vi "!DB_editor_Main.vi"(8 "error in (no error)":errorcluster, 11 "DB-editor in":refnum<class "DB-editor.lvclass">) -> (0 "error out":errorcluster, 3 "DB-editor out":refnum<class "DB-editor.lvclass">)   [LabVIEW 2020, in "Sgraph_lib_V1.lvlib" / "DB-editor.lvclass"]
doc: "Andre Koelewijn, 18 aug 2021\n\nDatabase properties editor application.\nOnly one instance of this VI should run, and only for administrative purposes.\n(only to be used to change settings)"
uses:
  DB-editor.lvclass
  Common/controls/typedef_com_TagProp.ctl
  FAMM/controls/Typedef_Gviewer_TagsUnits.ctl
  Gserver/controls/Typedef_QueryType.ctl
  DB-editor.lvclass/DB-editor.ctl
  Builds/Sgraph_lib_V1.lvlib
  FAMM/FAMM.lvclass
  Gserver/Gserver.lvclass
panel:
  in  "TAGprop":T1 {"TagFunc" format="%08x"; "RangeL" format="%.2f"; "RangeH" format="%.2f"}
  in  "Cancel":bool
  in  "Save":bool
  out "Qtype":string
  out "TAG":string
  in  "Ring":u16(ring)
  out "37x37":picture
  # "Database Editor"
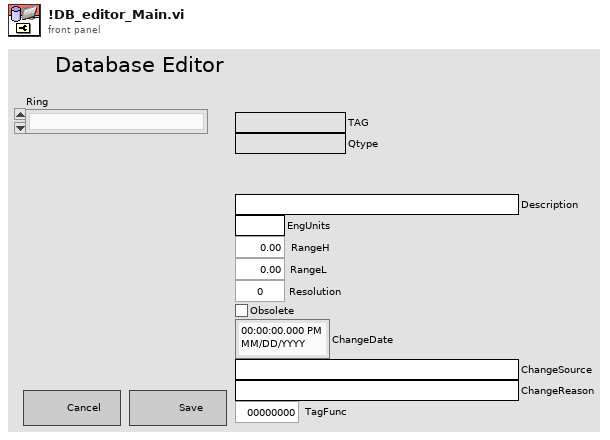
[diagram p1: front panel]
types:
  T1 = typedef "Sgraph_lib_V1.lvlib/typedef_com_TagProp.ctl" = cluster{"Description":string, "EngUnits":string, "RangeH":dbl, "RangeL":dbl, "Resolution":i32, "Obsolete":bool, "ChangeDate":timestamp, "ChangeSource":string, "ChangeReason":string, "TagFunc":u32}
  T2 = typedef "Sgraph_lib_V1.lvlib/FAMM.lvclass/Typedef_Gviewer_TagsUnits.ctl" = cluster{"PAQ_TAGs":string[], "WAQ_TAGs":string[], "EAQ_TAGs":string[], "PAQtagProps":T1[], "WAQtagProps":T1[], "EAQtagProps":T1[]}
  T3 = typedef "Sgraph_lib_V1.lvlib/Gserver.lvclass/Typedef_QueryType.ctl" = enum16{"Subscribe", "SubscribeNetw", "DataRequest", "RequestAllTags", "RequestIniPath", "FAMMstarted", "SetClientOptions", "GviewerUpdate", "OpenNewGraph", "CloseClient", "CloseAllClients", "Close Gserver", "OpenMemoryMap", "MeMapDataRequest", "MeMapDataResponse", "OpenDBeditor", "CheckDBeditorRunning", "StoppedDBeditor", "SaveDB_TAGpropRecord", "ConfirmDB_TAGpropSave", "GetXconstraints", "OpenNewNetworkGraph"}
  T4 = enum8{"Enabled", "Disabled", "Disabled and Grayed Out"}
  T5 = typedef "Typedef_Gserver-Replies.ctl" = cluster{"ServerActions":T6, "data":variant, "Source":string, "Time Stamp":timestamp}
  T6 = typedef "Sgraph_lib_V1.lvlib/Gviewer.lvclass/Typedef_ServerActions.ctl" = enum16{"GraphUpdate", "SendAllTags", "SendIniPath", "SetGeneralOptions", "EditTagsOpen", "EditTagsPresetSave", "EditTagsPresetLoad", "EditTagsClose", "NewTagSelection", "AutoScale", "DBeditStatus", "DBsaveConfirm", "GetXconstraints", "ExitGraph"}
  T7 = typedef "Sgraph_lib_V1.lvlib/DBAL.lvclass/DBAL_TAGprops.ctl" = T8[]
  T8 = typedef "Sgraph_lib_V1.lvlib/DBAL.lvclass/DBAL_TAGpropEdit.ctl" = cluster{"TAG":string, "Qtype":string, "TAGprop":T1}
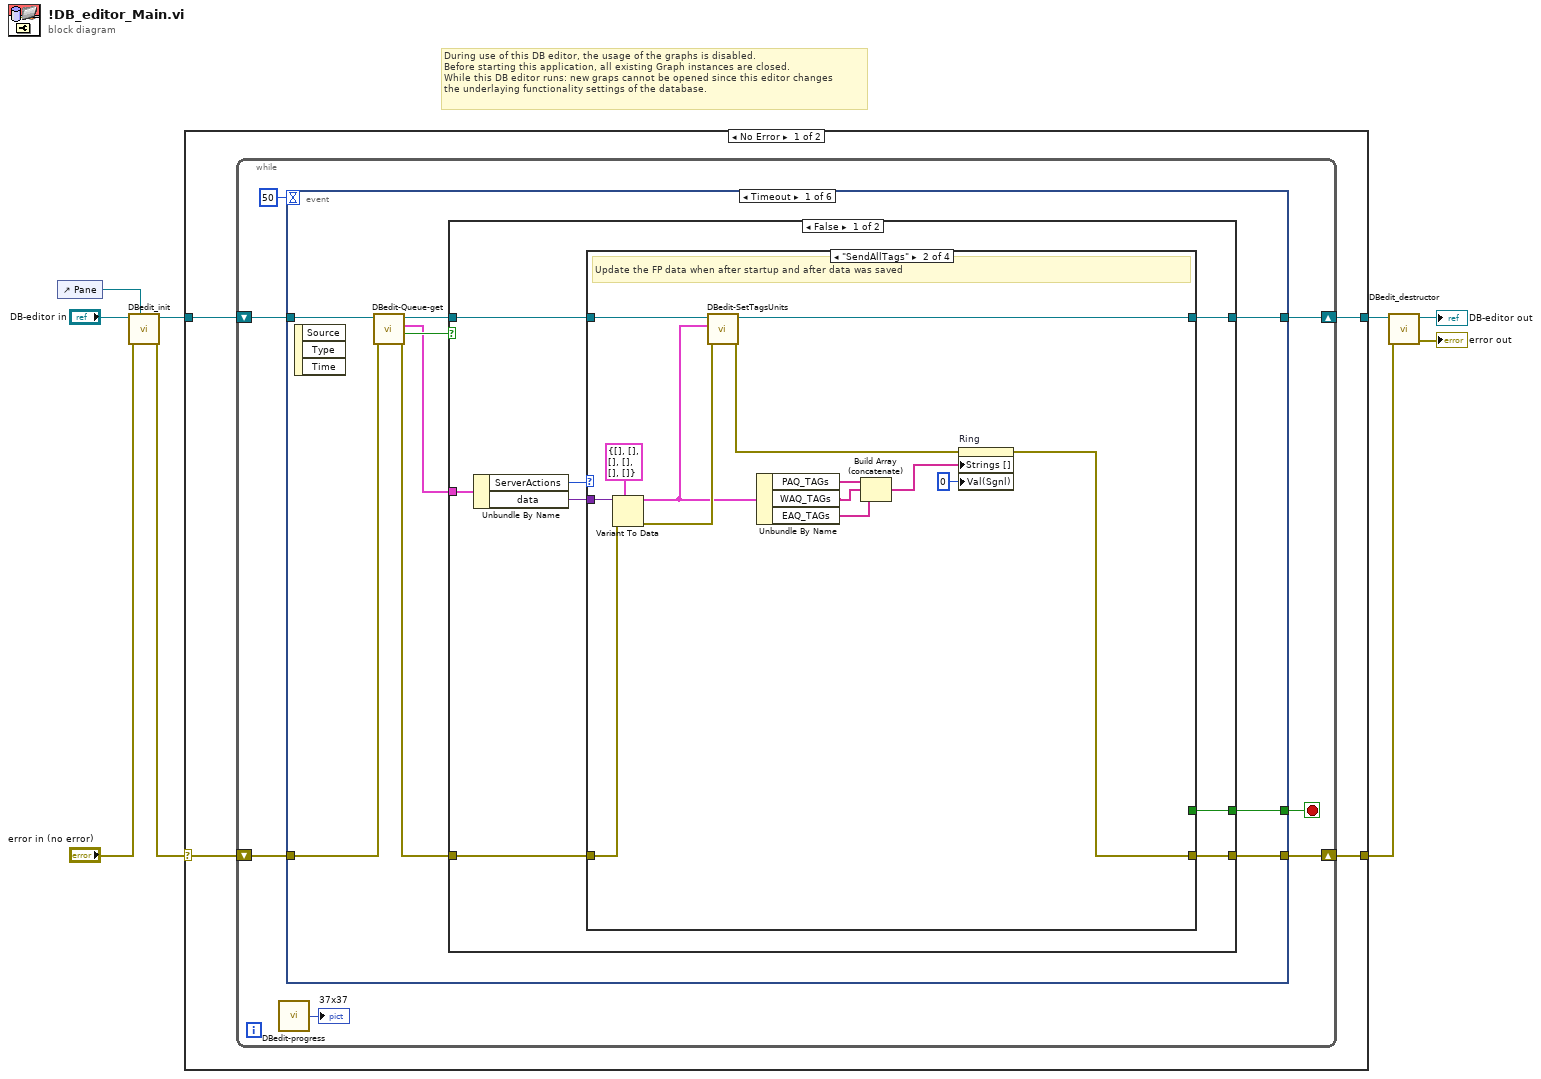
[diagram p0: block diagram]
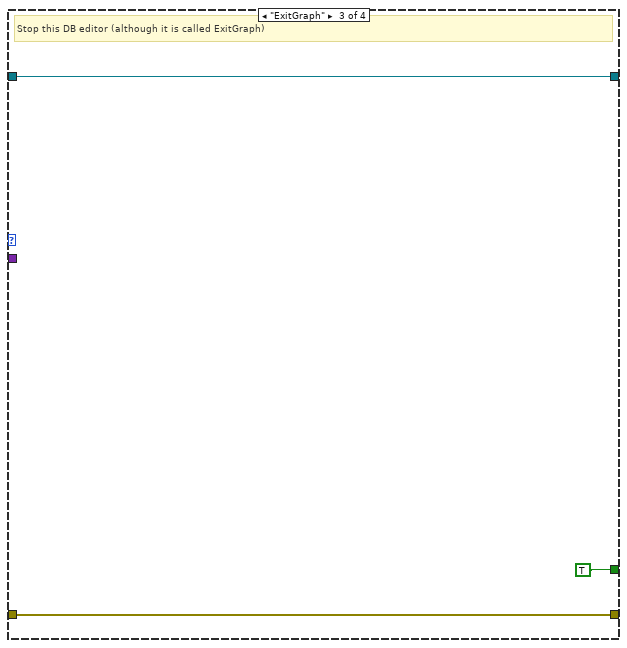
[diagram p3: hidden frame]
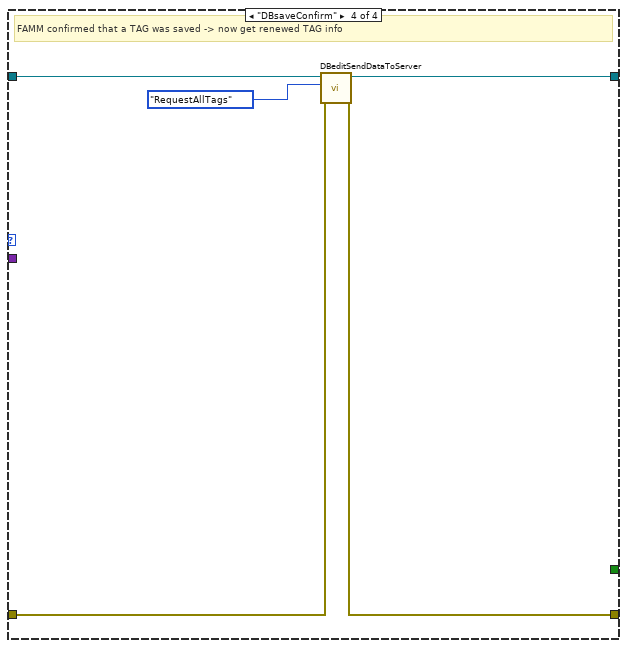
[diagram p4: hidden frame]
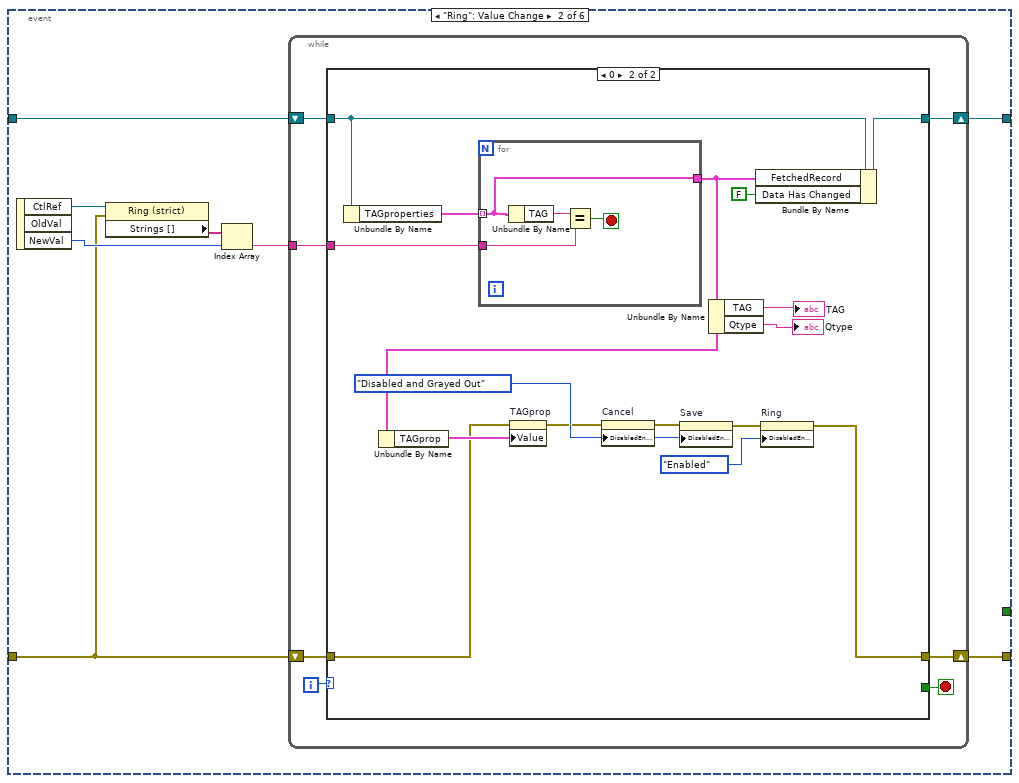
[diagram p6: hidden frame]
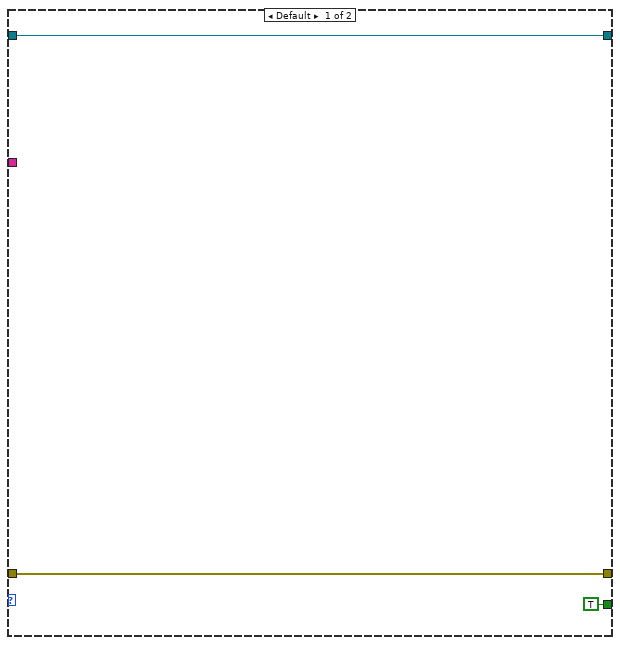
[diagram p7: hidden frame]
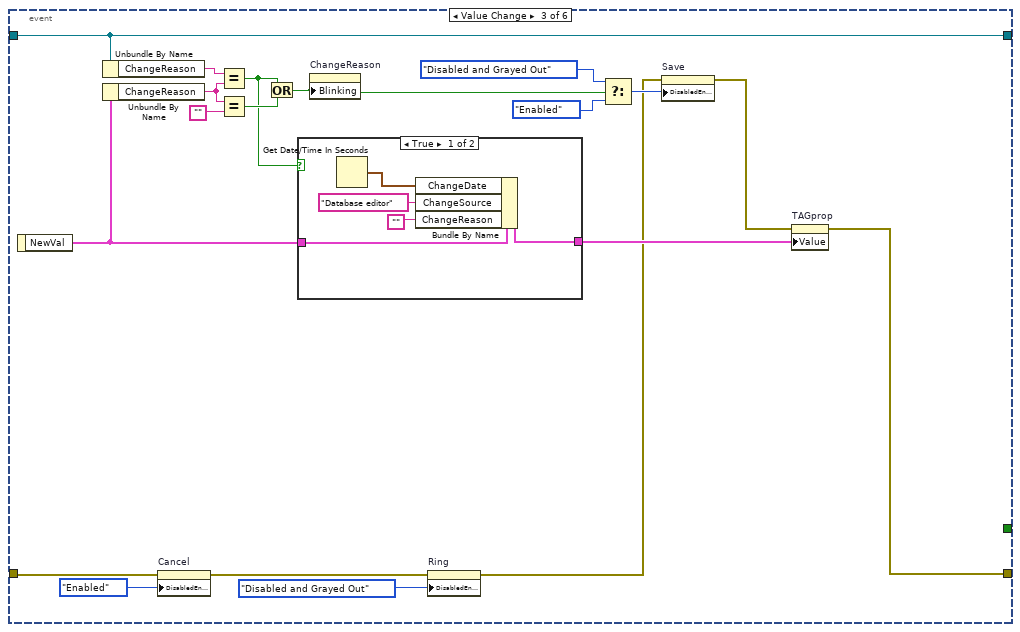
[diagram p8: hidden frame]
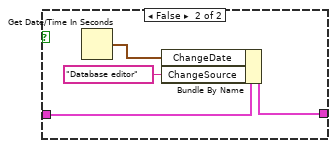
[diagram p9: hidden frame]
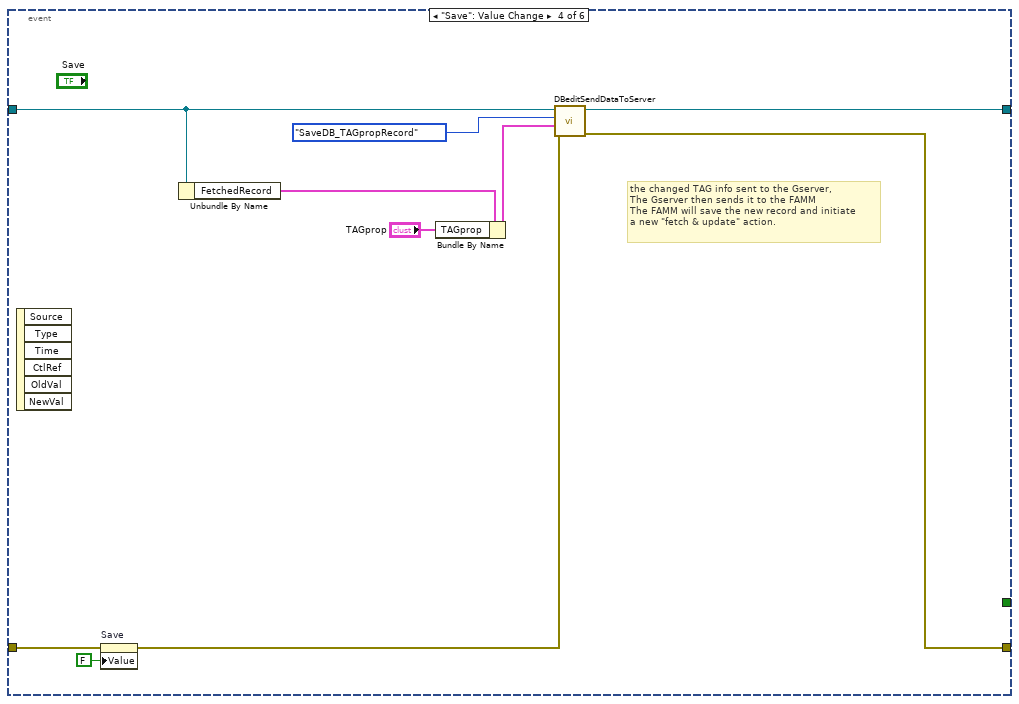
[diagram p10: hidden frame]
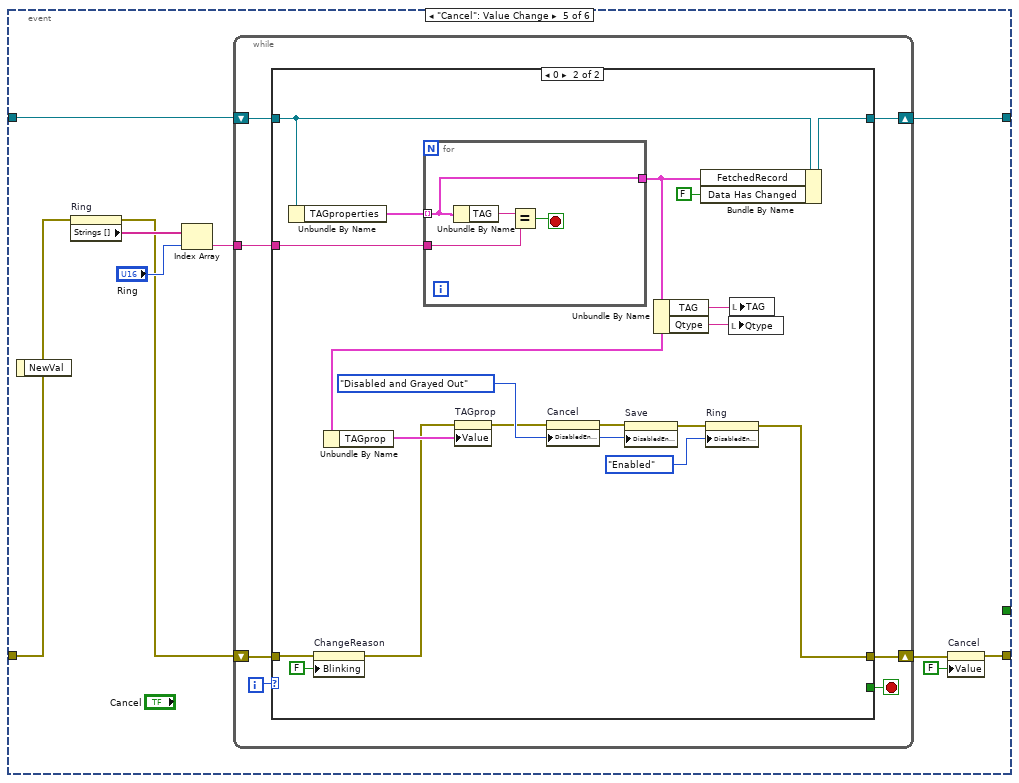
[diagram p11: hidden frame]
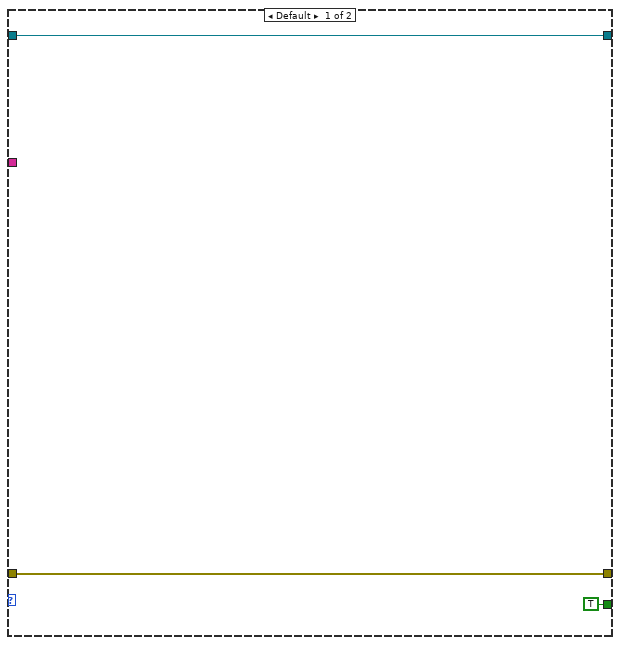
[diagram p12: hidden frame]
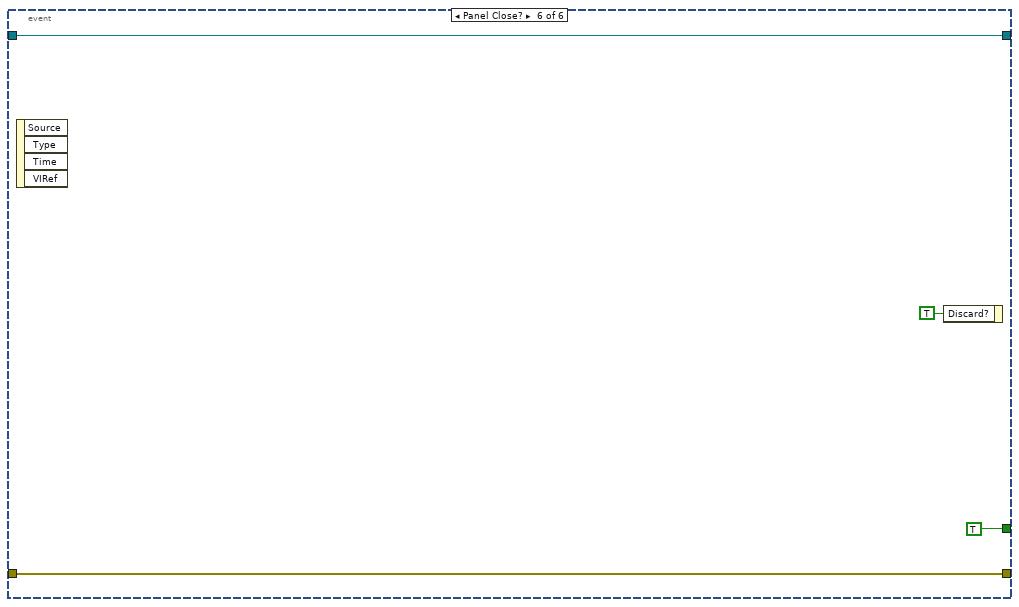
[diagram p13: hidden frame]
diagram:
  # "During use of this DB editor, the usage of the graphs is disabled.\nBefore starting this application, all existing Graph instances are closed.\nWhile this DB editor runs: new graps cannot be opened since this editor changes\nthe underlaying functionality settings of the database."
  n1 = control-ref of="Pane"() -> (w5:refnum<vi>)
  n2 = call "DBedit_init.vi"("Pane"=w5, "error in (no error)"="error in (no error)", "DB-editor in"="DB-editor in") -> ("error out"=w6:errorcluster, "DB-editor out"=w8:refnum<class "DB-editor.lvclass">)  [unwired: 7 in]
  n3 = case shown="No Error" w6 {
    selector: w6 -> [w12 w187]
    tunnel: [w10 w187] -> w2
    tunnel: [w11 w186] -> w4
    tunnel: w8 -> [w13 w186]
    frame No Error {
      n4 = while {
        shift-right: [w17] -> w11
        shift-left: w13 -> [w18]
        shift-right: [w19] -> w10
        shift-left: w12 -> [w20]
        stop <- w15 stop-if-true
        n5 = call "DBedit-progress.vi"() -> ("37x37"=→"37x37":picture)  [unwired: 6 in, 1 out]
        n6 = event shown="[0] Timeout" {
          selector: _ -> [_ _ _ _ _ _]
          dyn-events: _ -> [_ _ _ _ _ _]
          timeout: 50 -> [_ _ _ _ _ _]
          tunnel: w20 -> [w22 w67 w119 w137 w141 w183]
          tunnel: [w24 w65 w113 w130 w146 w183] -> w19
          tunnel: w18 -> [w29 w68 w117 w135 w145 w182]
          tunnel: [w25 w66 w117 w131 w140 w182] -> w17
          tunnel: [w21 _ _ _ _ TRUE] -> w15
          event Timeout {
            n7 = event-data() -> ()  [unwired: 1 in, 3 out]
            n8 = call "DBedit-Queue-get.vi"("error in (no error)"=w22, "Gviewer in"=w29) -> ("error out"=w23:errorcluster, "Time-out"=w28:bool, "Query"=w27:T5, "Gviewer out"=w26:refnum<class "DB-editor.lvclass">)  [unwired: 5 in, 1 out]
            n9 = case shown="False" w28 {
              tunnel: w27 -> [w37 _]
              tunnel: w26 -> [w35 w63]
              tunnel: [w34 w63] -> w25
              tunnel: w23 -> [w33 w62]
              tunnel: [w32 w62] -> w24
              tunnel: [w30 _] -> w21
              frame False {
                n10 = Unbundle By Name(w37) -> ("ServerActions"=w36:T6, "data"=w31:variant)
                n11 = case shown="\"SendAllTags\"" w36 {
                  tunnel: w35 -> [w38 w52 w56 w60]
                  tunnel: [w38 w53 w56 w59] -> w34
                  tunnel: w33 -> [w39 w49 w55 w58]
                  tunnel: [w39 w41 w55 w57] -> w32
                  tunnel: w31 -> [_ w51 _ _]
                  tunnel: [_ _ TRUE _] -> w30
                  frame Default {
                    # "Not implemented ..."
                  }
                  frame "SendAllTags" {
                    # "Update the FP data when after startup and after data was saved"
                    n12 = Variant To Data(error in=w49, type=T2 {"PAQ_TAGs"=[], "WAQ_TAGs"=[], "EAQ_TAGs"=[], "PAQtagProps"=[], "WAQtagProps"=[], "EAQtagProps"=[]} ("Tags_Units"), Variant=w51) -> (data=w47:T2, error out=w50:errorcluster)
                    n13 = call "DBedit-SetTagsUnits.vi"("error in (no error)"=w50, "Tags_Units"=w47, "Gviewer in"=w52) -> ("error out"=w42:errorcluster, "Gviewer out"=w53:refnum<class "DB-editor.lvclass">)  [unwired: 7 in]
                    n14 = Unbundle By Name(w47) -> ("PAQ_TAGs"=w46:string[], "WAQ_TAGs"=w45:string[], "EAQ_TAGs"=w44:string[])
                    n15 = Build Array (concatenate)(w46, w45, w44) -> (w43:string[])
                    n16 = property on="Ring" class="Ring (strict)"(error in=w42, "Strings []"=w43, "Val(Sgnl)"=u16 0 ("Value (Signaling)")) -> (error out=w41:errorcluster)  [unwired: 1 in, 1 out]
                  }
                  frame "ExitGraph" {
                    # "Stop this DB editor (although it is called ExitGraph)"
                  }
                  frame "DBsaveConfirm" {
                    # "FAMM confirmed that a TAG was saved -> now get renewed TAG info"
                    n17 = call "DBeditSendDataToServer.vi"("error in (no error)"=w58, "Query_type"=Typedef_QueryType."RequestAllTags", "Gviewer in"=w60) -> ("error out"=w57:errorcluster, "Gviewer out"=w59:refnum<class "DB-editor.lvclass">)  [unwired: 7 in]
                  }
                }
              }
              frame True {
              }
            }
          }
          event "Ring": Value Change {
            n18 = event-data() -> ("CtlRef"=w71:refnum<vi>, "NewVal"=w69:u16)  [unwired: 1 in, 1 out]
            n19 = property class="Ring (strict)"(reference=w71, error in=w67) -> ("Strings []"=w70:string[])  [unwired: 2 out]
            n20 = Index Array(array=w70, index=w69) -> (element=w64:string)
            n21 = while {
              shift-right: [w76] -> w66
              shift-left: w68 -> [w77]
              shift-right: [w74] -> w65
              shift-left: w67 -> [w75]
              tunnel: w64 -> [w72]
              i -> [w78]
              stop <- w73 stop-if-true
              n22 = case shown="0" w78 {
                tunnel: w77 -> [w81 w94]
                tunnel: [w81 w95] -> w76
                tunnel: w75 -> [w79 w85]
                tunnel: [w79 w82] -> w74
                tunnel: [TRUE _] -> w73
                tunnel: w72 -> [_ w96]
                frame Default {
                }
                frame 0 {
                  w88 = T4."Disabled and Grayed Out" ("Disabled")
                  n23 = Unbundle By Name(w94) -> ("TAGproperties"=w97:T7)
                  n24 = for {
                    tunnel: w97 -> [w98] mode=indexing
                    tunnel: w96 -> [w100]
                    tunnel: [w98] -> w90
                    stop <- w99 stop-if-true
                    n25 = Unbundle By Name(w98) -> ("TAG"=w101:string)
                    n26 = Equal?(x=w101, y=w100) -> (x = y?=w99:bool)
                  }
                  n27 = Unbundle By Name(w90) -> ("TAGprop"=w89:T1)
                  n28 = property on="TAGprop" class="Clust (strict)"(error in=w85, "Value"=w89) -> (error out=w87:errorcluster)  [unwired: 1 in, 1 out]
                  n29 = property on="Cancel" class="Bool (strict)"(error in=w87, "DisabledEnum"=w88) -> (error out=w86:errorcluster)  [unwired: 1 in, 1 out]
                  n30 = property on="Save" class="Bool (strict)"(error in=w86, "DisabledEnum"=w88) -> (error out=w83:errorcluster)  [unwired: 1 in, 1 out]
                  n31 = Unbundle By Name(w90) -> ("TAG"=→"TAG":string, "Qtype"=→"Qtype":string)
                  n32 = Bundle By Name(cluster=w94, "FetchedRecord"=w90, "Data Has Changed"=FALSE) -> (w95:refnum<class "DB-editor.lvclass">)
                  n33 = property on="Ring" class="Ring (strict)"(error in=w83, "DisabledEnum"=T4."Enabled" ("Disabled")) -> (error out=w82:errorcluster)  [unwired: 1 in, 1 out]
                }
              }
            }
          }
          event Value Change {
            n34 = event-data() -> ("NewVal"=w116:T1)  [unwired: 1 in]
            n35 = Unbundle By Name(w117) -> ("ChangeReason"=w115:string)
            n36 = Unbundle By Name(w116) -> ("ChangeReason"=w112:string)
            n37 = property on="Cancel" class="Bool (strict)"(error in=w119, "DisabledEnum"=T4."Enabled" ("Disabled")) -> (error out=w108:errorcluster)  [unwired: 1 in, 1 out]
            n38 = Equal?(x=w115, y=w112) -> (x = y?=w109:bool)
            n39 = Equal?(x=w112, y="") -> (x = y?=w110:bool)
            n40 = Or(x=w109, y=w110) -> (x .or. y?=w107:bool)
            n41 = case shown="True" w109 {
              tunnel: w116 -> [w125 w129]
              tunnel: [w122 w126] -> w114
              frame True {
                n42 = Get Date/Time In Seconds() -> (seconds since 1Jan1904=w124:timestamp)
                n43 = Bundle By Name(cluster=w125, "ChangeDate"=w124, "ChangeSource"="Database editor", "ChangeReason"="") -> (w122:T1)
              }
              frame False {
                n44 = Get Date/Time In Seconds() -> (seconds since 1Jan1904=w128:timestamp)
                n45 = Bundle By Name(cluster=w129, "ChangeDate"=w128, "ChangeSource"="Database editor") -> (w126:T1)
              }
            }
            n46 = property on="ChangeReason" class="Str"("Blinking"=w107) -> ()  [unwired: 2 in, 2 out]
            n47 = property on="Ring" class="Ring (strict)"(error in=w108, "DisabledEnum"=T4."Disabled and Grayed Out" ("Disabled")) -> (error out=w103:errorcluster)  [unwired: 1 in, 1 out]
            n48 = Select(t=T4."Disabled and Grayed Out" ("Disabled"), s=w107, f=T4."Enabled" ("Disabled")) -> (s? t:f=w104:T4)
            n49 = property on="Save" class="Bool (strict)"(error in=w103, "DisabledEnum"=w104) -> (error out=w102:errorcluster)  [unwired: 1 in, 1 out]
            n50 = property on="TAGprop" class="Clust (strict)"(error in=w102, "Value"=w114) -> (error out=w113:errorcluster)  [unwired: 1 in, 1 out]
          }
          event "Save": Value Change {
            # "the changed TAG info sent to the Gserver,\nThe Gserver then sends it to the FAMM\nThe FAMM will save the new record and initiate\na new \"fetch & update\" action."
            n51 = event-data() -> ()  [unwired: 1 in, 6 out]
            n52 = property on="Save" class="Bool (strict)"(error in=w137, "Value"=FALSE ("Save")) -> (error out=w138:errorcluster)  [unwired: 1 in, 1 out]
            n53 = Unbundle By Name(w135) -> ("FetchedRecord"=w134:T8)
            n54 = Bundle By Name(cluster=w134, "TAGprop"="TAGprop") -> (w132:T8)
            n55 = call "DBeditSendDataToServer.vi"("error in (no error)"=w138, "data"=w132, "Query_type"=Typedef_QueryType."SaveDB_TAGpropRecord", "Gviewer in"=w135) -> ("error out"=w130:errorcluster, "Gviewer out"=w131:refnum<class "DB-editor.lvclass">)  [unwired: 6 in]
          }
          event "Cancel": Value Change {
            n56 = event-data() -> ()  [unwired: 1 in, 1 out]
            n57 = property on="Ring" class="Ring (strict)"(error in=w141) -> (error out=w142:errorcluster, "Strings []"=w143:string[])  [unwired: 1 in, 1 out]
            n58 = Index Array(array=w143, index="Ring") -> (element=w148:string)
            n59 = while {
              shift-right: [w154] -> w140
              shift-left: w145 -> [w155]
              shift-right: [w152] -> w147
              shift-left: w142 -> [w153]
              tunnel: w148 -> [w150]
              i -> [w156]
              stop <- w151 stop-if-true
              n60 = case shown="0" w156 {
                tunnel: w155 -> [w159 w174]
                tunnel: [w159 w175] -> w154
                tunnel: w153 -> [w157 w162]
                tunnel: [w157 w165] -> w152
                tunnel: [TRUE _] -> w151
                tunnel: w150 -> [_ w176]
                frame Default {
                }
                frame 0 {
                  w170 = T4."Disabled and Grayed Out" ("Disabled")
                  n61 = Unbundle By Name(w174) -> ("TAGproperties"=w177:T7)
                  n62 = property on="ChangeReason" class="Str"(error in=w162, "Blinking"=FALSE) -> (error out=w160:errorcluster)  [unwired: 1 in, 1 out]
                  n63 = for {
                    tunnel: w177 -> [w178] mode=indexing
                    tunnel: w176 -> [w180]
                    tunnel: [w178] -> w172
                    stop <- w179 stop-if-true
                    n64 = Unbundle By Name(w178) -> ("TAG"=w181:string)
                    n65 = Equal?(x=w181, y=w180) -> (x = y?=w179:bool)
                  }
                  n66 = Unbundle By Name(w172) -> ("TAGprop"=w171:T1)
                  n67 = property on="TAGprop" class="Clust (strict)"(error in=w160, "Value"=w171) -> (error out=w169:errorcluster)  [unwired: 1 in, 1 out]
                  n68 = property on="Cancel" class="Bool (strict)"(error in=w169, "DisabledEnum"=w170) -> (error out=w168:errorcluster)  [unwired: 1 in, 1 out]
                  n69 = property on="Save" class="Bool (strict)"(error in=w168, "DisabledEnum"=w170) -> (error out=w166:errorcluster)  [unwired: 1 in, 1 out]
                  n70 = Unbundle By Name(w172) -> ("TAG"=w164:string, "Qtype"=w163:string)
                  n71 = Bundle By Name(cluster=w174, "FetchedRecord"=w172, "Data Has Changed"=FALSE) -> (w175:refnum<class "DB-editor.lvclass">)
                  n72 = property on="Ring" class="Ring (strict)"(error in=w166, "DisabledEnum"=T4."Enabled" ("Disabled")) -> (error out=w165:errorcluster)  [unwired: 1 in, 1 out]
                  n73 = local write "Qtype"(w163) -> ()
                  n74 = local write "TAG"(w164) -> ()
                }
              }
            }
            n75 = property on="Cancel" class="Bool (strict)"(error in=w147, "Value"=FALSE ("Cancel")) -> (error out=w146:errorcluster)  [unwired: 1 in, 1 out]
          }
          event Panel Close? {
            n76 = event-data() -> ()  [unwired: 1 in, 4 out]
            n77 = event-data("Discard?"=TRUE) -> ()  [unwired: 1 in, 1 out]
          }
        }
      }
    }
    frame Error {
    }
  }
  n78 = call "DBedit_destructor.vi"("error in (no error)"=w2, "DB-editor in"=w4) -> ("error out"=→"error out":errorcluster, "DB-editor out"=→"DB-editor out":refnum<class "DB-editor.lvclass">)  [unwired: 8 in]
